vi "Close MeasurementLink Session.vi"(8 "error in":errorcluster, 9 "initialize and close session behavior":T1, 10 "session in":variant, 11 "session factory in":refnum<class "Session Factory.lvclass">) -> (0 "error out":errorcluster)   [LabVIEW 2020, in "IVI Scope Instrument.lvlib" / "Session Factory.lvclass"]
doc: "Closes the local session. If the session represents a remote session, <b>initialize and close session behavior</b> determines whether closing the local session closes the server session or detaches from the server session."
uses:
  Session Factory.lvclass
  <vilib>/MeasurementLink/MeasurementLink Instrument/ISession Factory/Initialize and Close Session Behavior.ctl
  <vilib>/MeasurementLink/MeasurementLink Instrument/ISession Factory/ISession Factory.lvclass
  <vilib>/ivi/iviscope/_iviscope.llb/IviScope Close.vi
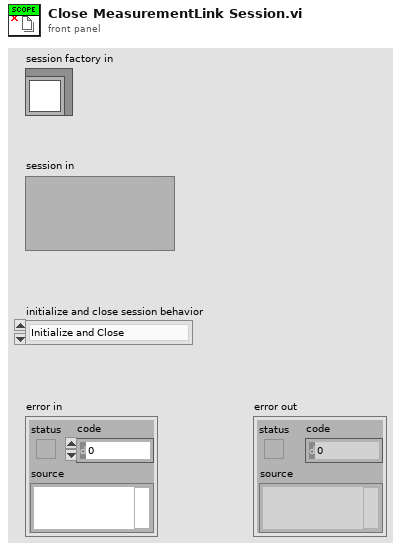
[diagram p1: front panel]
types:
  T1 = typedef "MeasurementLink Instrument.lvlib/ISession Factory.lvclass/Initialize and Close Session Behavior.ctl" = enum16{"Initialize and Close", "Attach and Detach", "Initialize and Detach", "Attach and Close"}
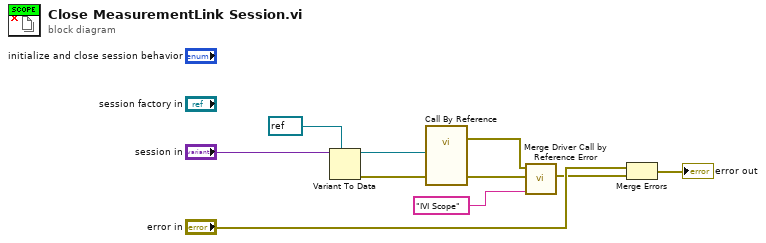
[diagram p0: block diagram]
diagram:
  n1 = Variant To Data(type=refnum<k15> refnum ("instrument handle"), Variant="session in") -> (data=w9:refnum<k15>, error out=w6:errorcluster)  [unwired: 1 in]
  n2 = call-by-ref "?"("error in (no error)"=w6, "instrument handle"=w9) -> (error out=w4:errorcluster, 0:"error out"=w5:errorcluster)  [unwired: 11 in, 1 out]
  n3 = call <vilib>:"Merge Driver Call by Reference Error.vi"("driver name"="IVI Scope", "called vi error"=w5, "call by ref error"=w4) -> ("error out"=w2:errorcluster)  [unwired: 8 in]
  n4 = Merge Errors("error in", w2) -> (→"error out":errorcluster)
